vi "Write signal out.vi"(8 "error in (no error)":errorcluster, 10 "signal out":waveform(dbl)(graph)={"t0"=timestamp(3020748.0 s since 1904-01-01), "dt"=0.001, "Y"=array[1000 elements]}, 11 "SignalIn in":refnum<class "SignalIn.lvclass">) -> (0 "error out":errorcluster, 3 "SignalIn out":refnum<class "SignalIn.lvclass">)   [LabVIEW 2011, in "SignalIn.lvclass"]
uses:
  SignalIn.lvclass
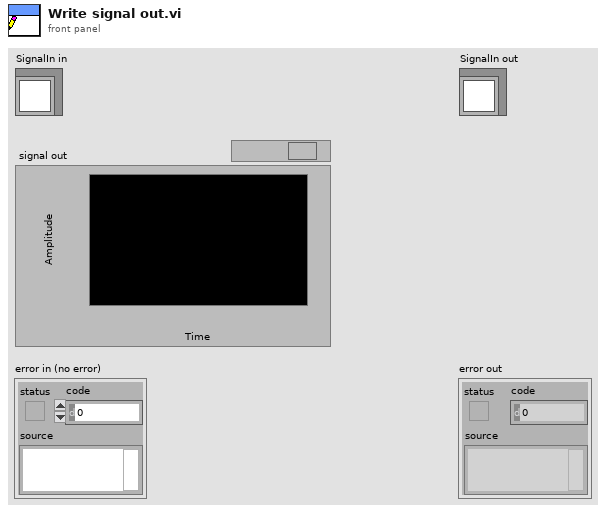
[diagram p1: front panel]
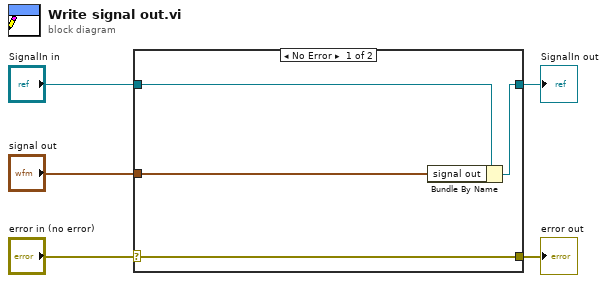
[diagram p0: block diagram]
diagram:
  n1 = case shown="No Error" "error in (no error)" {
    selector: "error in (no error)" -> [w9 w10]
    tunnel: [w9 w10] -> w4
    tunnel: [w7 w11] -> w2
    tunnel: "SignalIn in" -> [w8 w11]
    tunnel: "signal out" -> [w6 _]
    frame No Error {
      n2 = Bundle By Name(cluster=w8, "signal out"=w6) -> (w7:refnum<class "SignalIn.lvclass">)
    }
    frame Error {
    }
  }
  "error out" <- w4
  "SignalIn out" <- w2
